vi "Source_Q_wrong.vi"(2 "Ch Names":string[](array[string]), 3 "Values":dbl[](array[numeric]) format="%.2f") -> (0 "Gas Error?":bool)   [LabVIEW 2013]
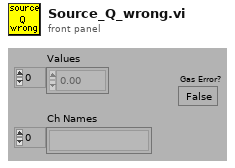
[diagram p1: front panel]
types:
  T1 = enum16{"Append to Global", "Read Global then Clear"}
  T2 = typedef "Ch_description_ADAM.ctl" = cluster{"Ch Name":string, "Type":T3, "Function":T4, "Ch State":T5, "Calibration type":T6, "A":dbl, "B":dbl, "C":dbl, "D":dbl, "Comments":string, "Address":T7, "String":string, "Duty":u16}
  T3 = typedef "Module_type_ADAM.ctl" = string
  T4 = typedef "Function_ADAM.ctl" = enum16{"Analogue Input", "Digital Input", "Event counter", "Event rate", "Analogue Output", "Digital Output", "Relay Output"}
  T5 = typedef "Channel_State.ctl" = enum16{"On", "Off", "Always On", "Always Off"}
  T6 = typedef "Calib_type_ADAM.ctl" = enum16{"Raw", "Bx + A", "Cx^2 + Bx + A", "Dx^3 + Cx^2 + Bx + A", "In Band", "Hi-Tec Q", "Hi-Tec M_dot", "Text"}
  T7 = typedef "Address.ctl" = cluster{"Main":i32, "Ch.":i32, "Sub":i32, "Port Name":string}
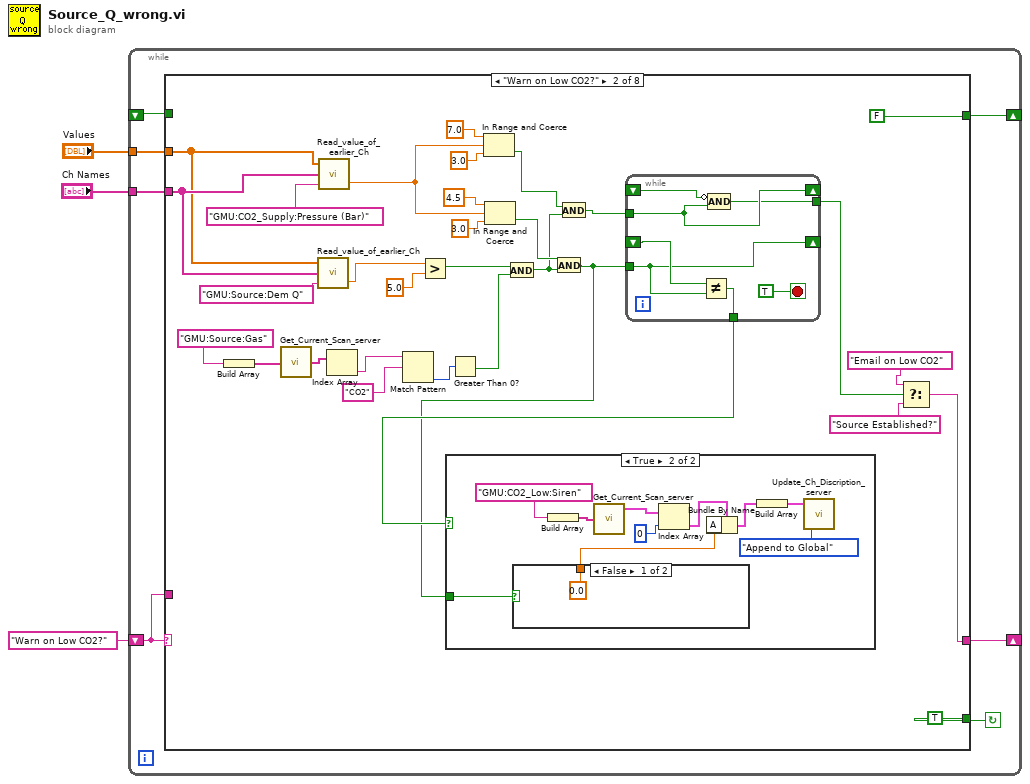
[diagram p0: block diagram]
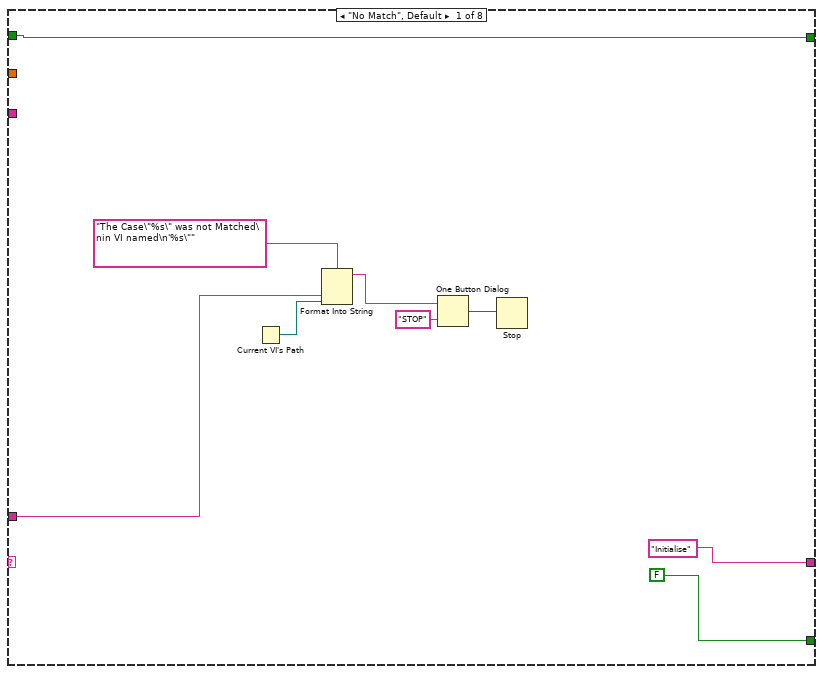
[diagram p2: hidden frame]
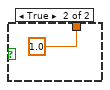
[diagram p4: hidden frame]
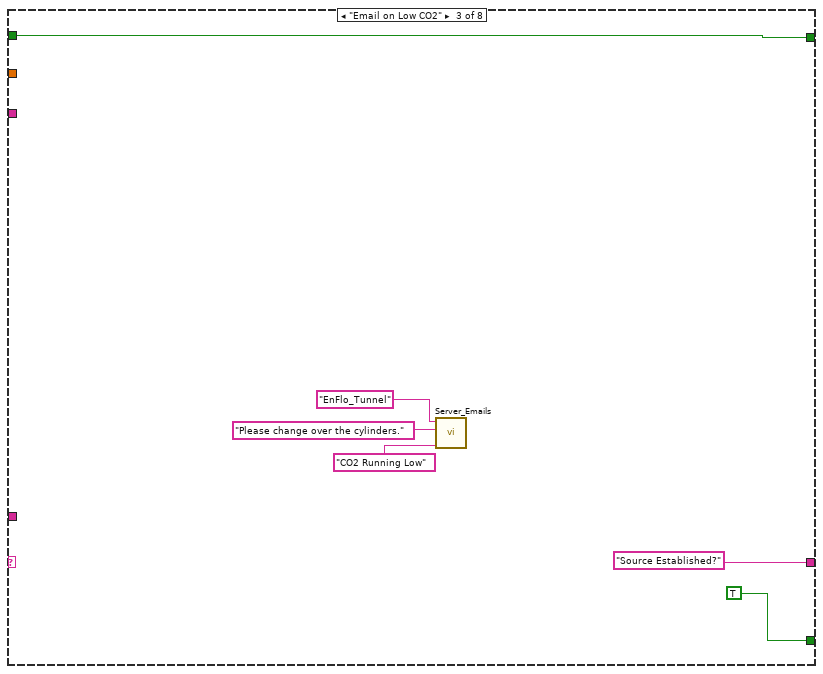
[diagram p5: hidden frame]
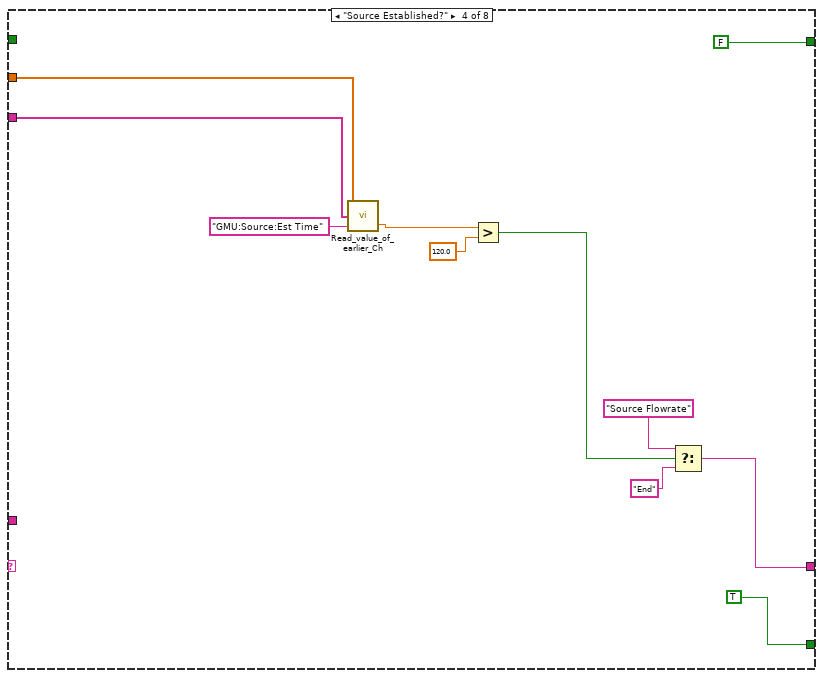
[diagram p6: hidden frame]
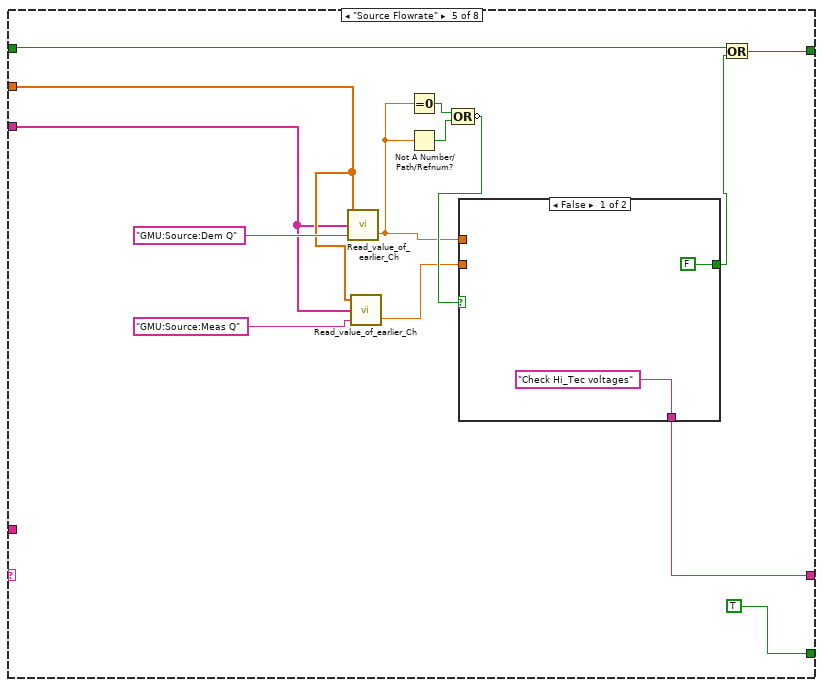
[diagram p7: hidden frame]
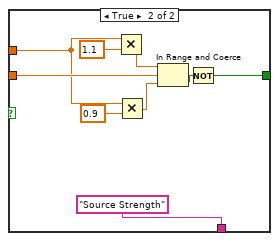
[diagram p8: hidden frame]
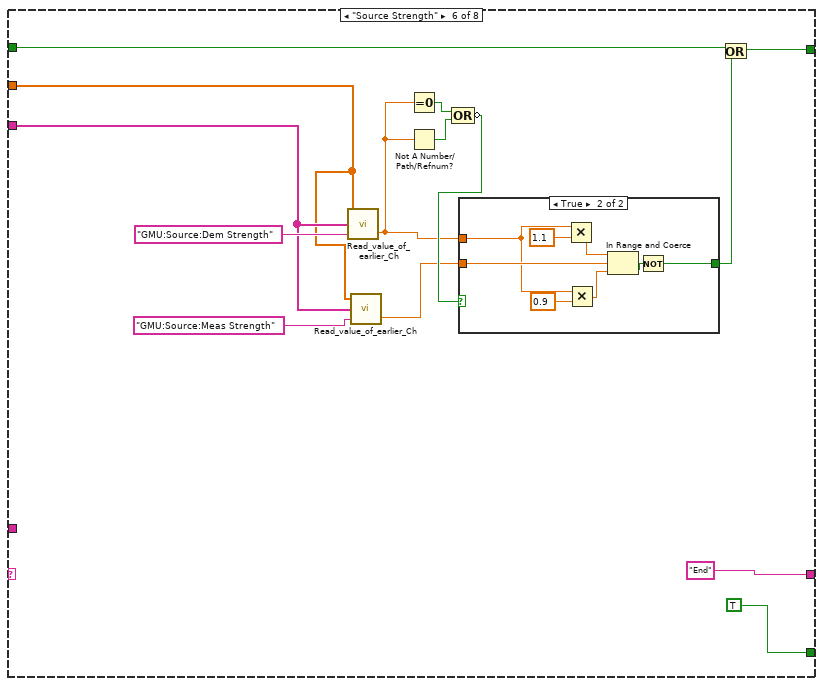
[diagram p9: hidden frame]
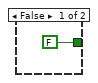
[diagram p10: hidden frame]
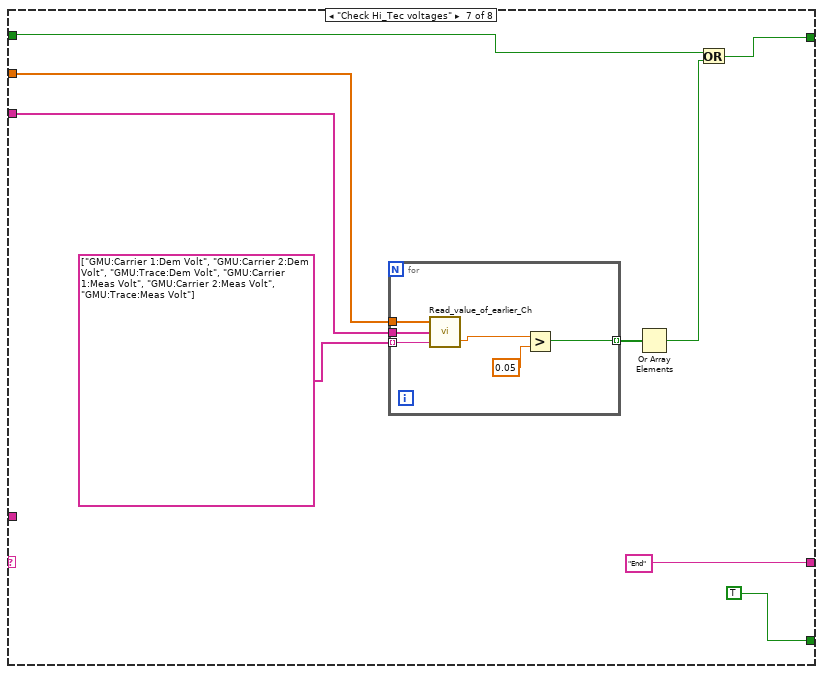
[diagram p11: hidden frame]
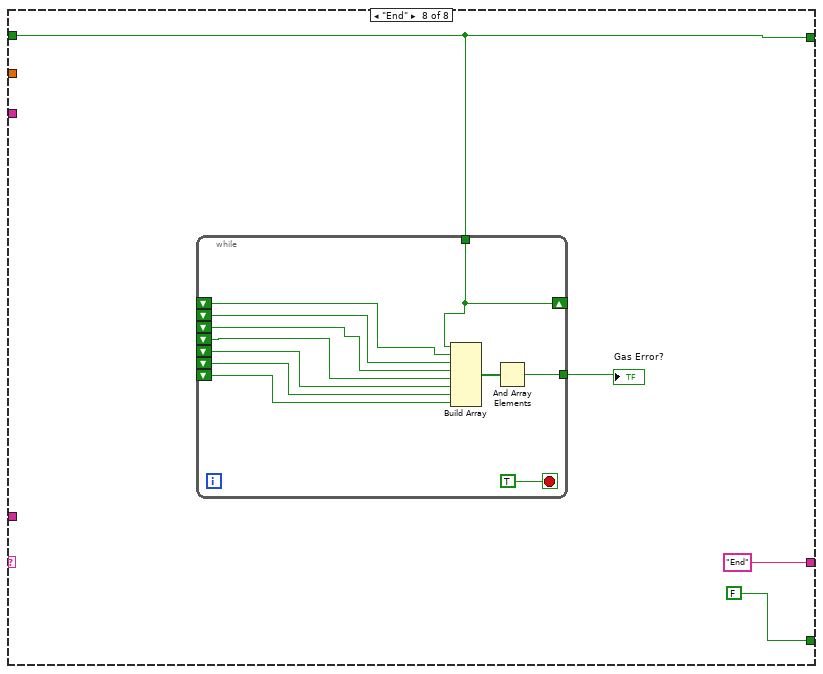
[diagram p12: hidden frame]
diagram:
  n1 = while {
    shift-left: "Warn on Low CO2?" -> [w8]
    shift-right: [w9] -> _
    tunnel: "Ch Names" -> [w7]
    tunnel: "Values" -> [w6]
    shift-right: [w5] -> _
    shift-left: _ -> [w4]
    stop <- w10 continue-if-true
    n2 = case shown="\"Warn on Low CO2?\"" w8 {
      tunnel: [FALSE TRUE TRUE TRUE TRUE TRUE TRUE FALSE] -> w10
      tunnel: ["Initialise" w21 "Source Established?" w77 w87 "End" ("f") "End" "End" ("f")] -> w9
      tunnel: w8 -> [w14 _ _ _ _ _ _ _]
      tunnel: w7 -> [_ w44 _ w85 w98 w114 w141 _]
      tunnel: w6 -> [_ w43 _ w84 w99 w113 w139 _]
      tunnel: [w11 FALSE w74 FALSE w90 w115 w135 w151] -> w5
      tunnel: w4 -> [w11 _ w74 _ w88 w116 w136 w151]
      frame "No Match", Default {
        n3 = Current VI's Path() -> (path=w13:path)
        n4 = Format Into String(format string="The Case\"%s\" was not Matched\nin VI named\n'%s\"" ("Format String"), w14, w13) -> (resulting string=w17:string)  [unwired: 2 in, 1 out]
        n5 = One Button Dialog(message=w17, button name ("OK")="STOP") -> (true=w15:bool)
        n6 = Stop(stop? (T)=w15) -> ()
      }
      frame "Warn on Low CO2?" {
        n7 = Build Array("GMU:Source:Gas") -> (w38:string[])
        n8 = call "Get_Current_Scan_server.vi"("Desired Channels"=w38) -> ("String values"=w37:string[])  [unwired: 2 out]
        n9 = call "Read_value_of_earlier_Ch.vi"("Desired Ch to Read"="GMU:Source:Dem Q", "Ch names"=w44, "Present scan array"=w43) -> ("Value"=w42:dbl)  [unwired: 1 in, 1 out]
        n10 = call "Read_value_of_earlier_Ch.vi"("Desired Ch to Read"="GMU:CO2_Supply:Pressure (Bar)", "Ch names"=w44, "Present scan array"=w43) -> ("Value"=w31:dbl)  [unwired: 1 in, 1 out]
        n11 = Index Array(array=w37) -> (element=w36:string)  [unwired: 1 in]
        n12 = Match Pattern(string=w36, regular expression="CO2") -> (offset past match=w34:i32)  [unwired: 1 in, 3 out]
        n13 = Greater?(x=w42, y=5.0) -> (0:w30:bool)
        n14 = Greater Than 0?(x=w34) -> (x > 0?=w29:bool)
        n15 = In Range and Coerce(upper limit=7.0, x=w31, lower limit=3.0) -> (In Range?=w28:bool)  [unwired: 1 out]
        n16 = In Range and Coerce(upper limit=4.5, x=w31, lower limit=3.0) -> (In Range?=w27:bool)  [unwired: 1 out]
        n17 = And(x=w30, y=w29) -> (x .and. y?=w25:bool)
        n18 = And(x=w27, y=w25) -> (x .and. y?=w26:bool)
        n19 = And(x=w28, y=w25) -> (x .and. y?=w24:bool)
        n20 = while {
          shift-right: [w67] -> _
          shift-left: _ -> [w68]
          tunnel: w26 -> [w67]
          tunnel: [w66] -> w40
          shift-right: [w65] -> _
          shift-left: _ -> [w64]
          tunnel: w24 -> [w65]
          tunnel: [w63] -> w23
          stop <- TRUE stop-if-true
          n21 = Not Equal?(x=w68, y=w67) -> (x != y?=w66:bool)
          n22 = Compound Arithmetic op=AND(invert w64, w65) -> (w63:bool)
        }
        n23 = case shown="True" w40 {
          tunnel: w26 -> [_ w59]
          frame False {
          }
          frame True {
            n24 = case shown="False" w59 {
              tunnel: [0.0 ("A") 1.0 ("A")] -> w54
              frame False {
              }
              frame True {
              }
            }
            n25 = Build Array("GMU:CO2_Low:Siren") -> (w58:string[])
            n26 = call "Get_Current_Scan_server.vi"("Desired Channels"=w58) -> ("Ch Description Array"=w57:T2[])  [unwired: 2 out]
            n27 = Index Array(array=w57, index=0) -> (element=w55:T2)
            n28 = Bundle By Name(cluster=w55, "A"=w54) -> (w52:T2)
            n29 = Build Array(w52) -> (w51:T2[])
            n30 = call "Update_Ch_Discription_server.vi"("Mode"=T1."Append to Global", "Channels to update In"=w51) -> ()  [unwired: 1 in, 1 out]
          }
        }
        n31 = Select(t="Email on Low CO2", s=w23, f="Source Established?") -> (s? t:f=w21:string)
      }
      frame "Email on Low CO2" {
        n32 = call "Server_Emails.vi"("Client Name Contains"="EnFlo_Tunnel", "Message"="Please change over the cylinders.", "Subject"="CO2 Running Low") -> ()  [unwired: 2 in, 3 out]
      }
      frame "Source Established?" {
        n33 = call "Read_value_of_earlier_Ch.vi"("Desired Ch to Read"="GMU:Source:Est Time", "Ch names"=w85, "Present scan array"=w84) -> ("Value"=w82:dbl)  [unwired: 1 in, 1 out]
        n34 = Greater?(x=w82, y=120.0) -> (0:w79:bool)
        n35 = Select(t="Source Flowrate", s=w79, f="End") -> (s? t:f=w77:string)
      }
      frame "Source Flowrate" {
        n36 = call "Read_value_of_earlier_Ch.vi"("Desired Ch to Read"="GMU:Source:Dem Q", "Ch names"=w98, "Present scan array"=w99) -> ("Value"=w93:dbl)  [unwired: 1 in, 1 out]
        n37 = call "Read_value_of_earlier_Ch.vi"("Desired Ch to Read"="GMU:Source:Meas Q", "Ch names"=w98, "Present scan array"=w99) -> ("Value"=w92:dbl)  [unwired: 1 in, 1 out]
        n38 = Equal To 0?(x=w93) -> (x = 0?=w96:bool)
        n39 = Not A Number/Path/Refnum?(number/path/refnum=w93) -> (NaN/Path/Refnum?=w95:bool)
        n40 = Compound Arithmetic op=OR(w96, w95) -> (invert w94:bool)
        n41 = case shown="False" w94 {
          tunnel: w92 -> [_ w107]
          tunnel: w93 -> [_ w106]
          tunnel: [FALSE w104] -> w89
          tunnel: ["Check Hi_Tec voltages" "Source Strength"] -> w87
          frame False {
          }
          frame True {
            n42 = Multiply(x=w106, y=1.1) -> (x*y=w111:dbl)
            n43 = Multiply(x=w106, y=0.9) -> (x*y=w110:dbl)
            n44 = In Range and Coerce(upper limit=w111, x=w107, lower limit=w110) -> (In Range?=w105:bool)  [unwired: 1 out]
            n45 = Not(x=w105) -> (.not. x?=w104:bool)
          }
        }
        n46 = Or(x=w88, y=w89) -> (x .or. y?=w90:bool)
      }
      frame "Source Strength" {
        n47 = call "Read_value_of_earlier_Ch.vi"("Desired Ch to Read"="GMU:Source:Dem Strength", "Ch names"=w114, "Present scan array"=w113) -> ("Value"=w120:dbl)  [unwired: 1 in, 1 out]
        n48 = call "Read_value_of_earlier_Ch.vi"("Desired Ch to Read"="GMU:Source:Meas Strength", "Ch names"=w114, "Present scan array"=w113) -> ("Value"=w119:dbl)  [unwired: 1 in, 1 out]
        n49 = Equal To 0?(x=w120) -> (x = 0?=w123:bool)
        n50 = Not A Number/Path/Refnum?(number/path/refnum=w120) -> (NaN/Path/Refnum?=w122:bool)
        n51 = Compound Arithmetic op=OR(w123, w122) -> (invert w121:bool)
        n52 = case shown="True" w121 {
          tunnel: w119 -> [_ w130]
          tunnel: w120 -> [_ w129]
          tunnel: [FALSE w127] -> w117
          frame False {
          }
          frame True {
            n53 = Multiply(x=w129, y=1.1) -> (x*y=w134:dbl)
            n54 = Multiply(x=w129, y=0.9) -> (x*y=w133:dbl)
            n55 = In Range and Coerce(upper limit=w134, x=w130, lower limit=w133) -> (In Range?=w128:bool)  [unwired: 1 out]
            n56 = Not(x=w128) -> (.not. x?=w127:bool)
          }
        }
        n57 = Or(x=w116, y=w117) -> (x .or. y?=w115:bool)
      }
      frame "Check Hi_Tec voltages" {
        n58 = for {
          tunnel: w139 -> [w149]
          tunnel: w141 -> [w148]
          tunnel: string[] ["GMU:Carrier 1:Dem Volt", "GMU:Carrier 2:Dem Volt", "GMU:Trace:Dem Volt", "GMU:Carrier 1:Meas Volt", "GMU:Carrier 2:Meas Volt", "GMU:Trace:Meas Volt"] ("appended array") -> [w147] mode=indexing
          tunnel: [w144] -> w138 mode=indexing
          n59 = call "Read_value_of_earlier_Ch.vi"("Desired Ch to Read"=w147, "Ch names"=w148, "Present scan array"=w149) -> ("Value"=w145:dbl)  [unwired: 1 in, 1 out]
          n60 = Greater?(x=w145, y=0.05) -> (0:w144:bool)
        }
        n61 = Or Array Elements(Boolean array=w138) -> (logical OR=w137:bool)
        n62 = Or(x=w136, y=w137) -> (x .or. y?=w135:bool)
      }
      frame "End" {
        n63 = while {
          shift-right: [w163] -> _
          shift-left: _ -> [w162]
          shift-left: _ -> [w161]
          shift-left: _ -> [w160]
          shift-left: _ -> [w159]
          shift-left: _ -> [w158]
          shift-left: _ -> [w157]
          shift-left: _ -> [w156]
          tunnel: w151 -> [w163]
          tunnel: [w154] -> w153
          stop <- TRUE stop-if-true
          n64 = Build Array(w163, w162, w161, w160, w159, w158, w157, w156) -> (w155:bool[])
          n65 = And Array Elements(Boolean array=w155) -> (logical AND=w154:bool)
        }
        "Gas Error?" <- w153
      }
    }
  }
